vi "Non-zero increment min max.vi"(11 "Data":dbl[](array[numeric])) -> (2 "max value":dbl, 3 "min value":dbl)   [LabVIEW 2016]
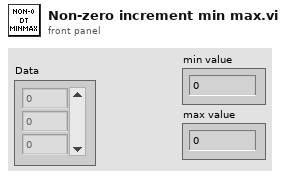
[diagram p1: front panel]
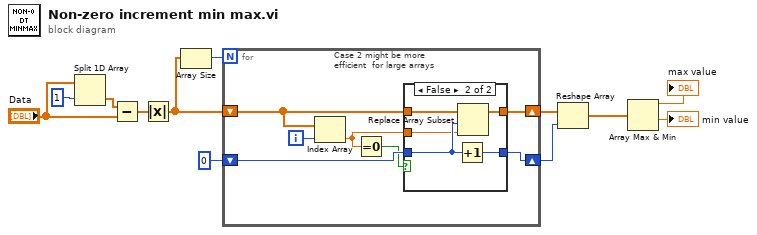
[diagram p0: block diagram]
diagram:
  n1 = Split 1D Array(array="Data", index=1) -> (second subarray=w11:dbl[])  [unwired: 1 out]
  n2 = Subtract(x=w11, y="Data") -> (x-y=w9:dbl[])
  n3 = Absolute Value(x=w9) -> (abs(x)=w4:dbl[])
  n4 = Array Size(array=w4) -> (size(s)=w8:i32)
  n5 = for {
    N: w8 -> [_]
    shift-right: [w19] -> w6
    shift-left: w4 -> [w17]
    shift-right: [w15] -> w5
    shift-left: 0 -> [w16]
    i -> [w18]
    # "Case 2 might be more\nefficient  for large arrays"
    n6 = Index Array(array=w17, index=w18) -> (element=w13:dbl)
    n7 = Equal To 0?(x=w13) -> (x = 0?=w14:bool)
    n8 = case shown="False" w14 {
      tunnel: w17 -> [w21 w26]
      tunnel: [w21 w25] -> w19
      tunnel: w16 -> [w20 w24]
      tunnel: [w20 w23] -> w15
      tunnel: w13 -> [_ w22]
      frame True {
      }
      frame False {
        n9 = Increment(x=w24) -> (x+1=w23:i32)
        n10 = Replace Array Subset(array=w26, new element=w22, index=w24) -> (w25:dbl[])
      }
    }
  }
  n11 = Reshape Array(w6, w5) -> (w3:dbl[])
  n12 = Array Max & Min(array=w3) -> (max value=→"max value":dbl, min value=→"min value":dbl)  [unwired: 2 out]
